vi "Cost Calculation.vi"(5 "Weights":T1={"TS-S weight"=90.0, "CS-S weight"=90.0, "PCS-S weight"=90.0, "Near weight"=90.0, "Mid weight"=90.0, "Far weight"=90.0}, 7 "Previous Calculated Sector":i16=90, 8 "Far Boolean Array":bool[](array[boolean]), 9 "Mid Boolean Array":bool[](array[boolean]), 10 "Near Boolean Array":bool[](array[boolean]), 11 "Target Sector":i16=90) -> (3 "Cost Array":dbl[](array[numeric]))   [LabVIEW 2009]
uses:
  VFH Weights.ctl
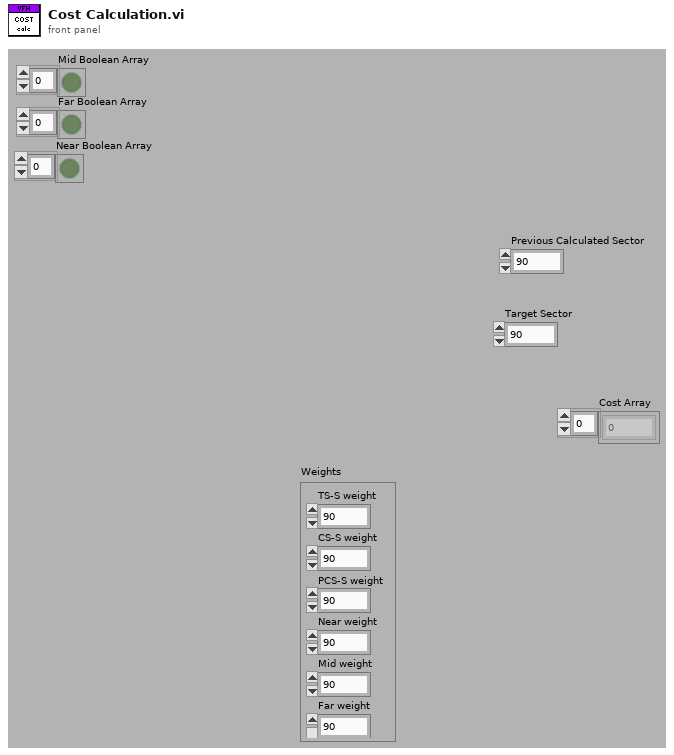
[diagram p1: front panel]
types:
  T1 = typedef "VFH Weights.ctl" = cluster{"TS-S weight":dbl, "CS-S weight":dbl, "PCS-S weight":dbl, "Near weight":dbl, "Mid weight":dbl, "Far weight":dbl}
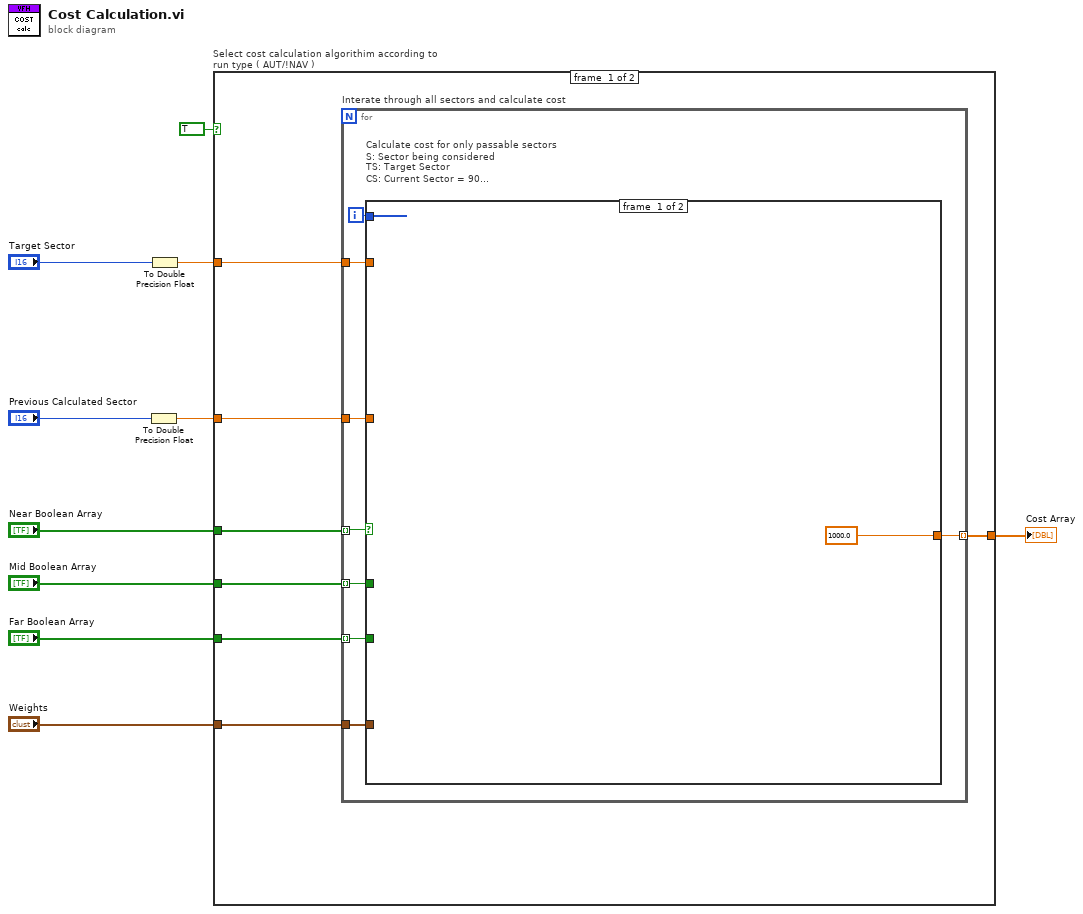
[diagram p0: block diagram]
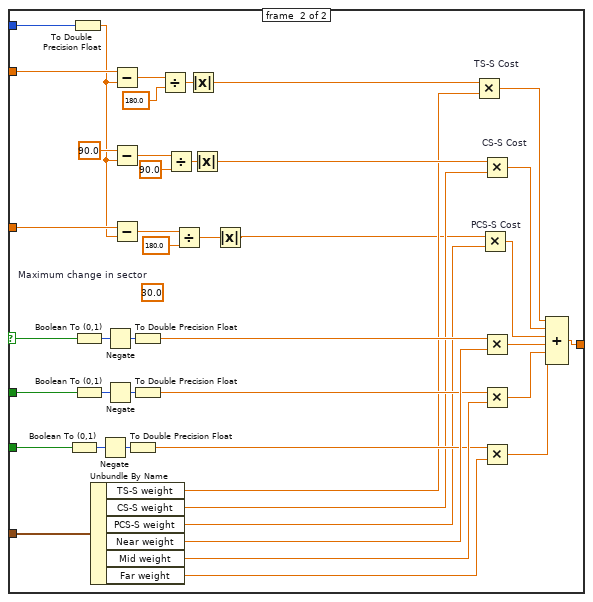
[diagram p2: hidden frame]
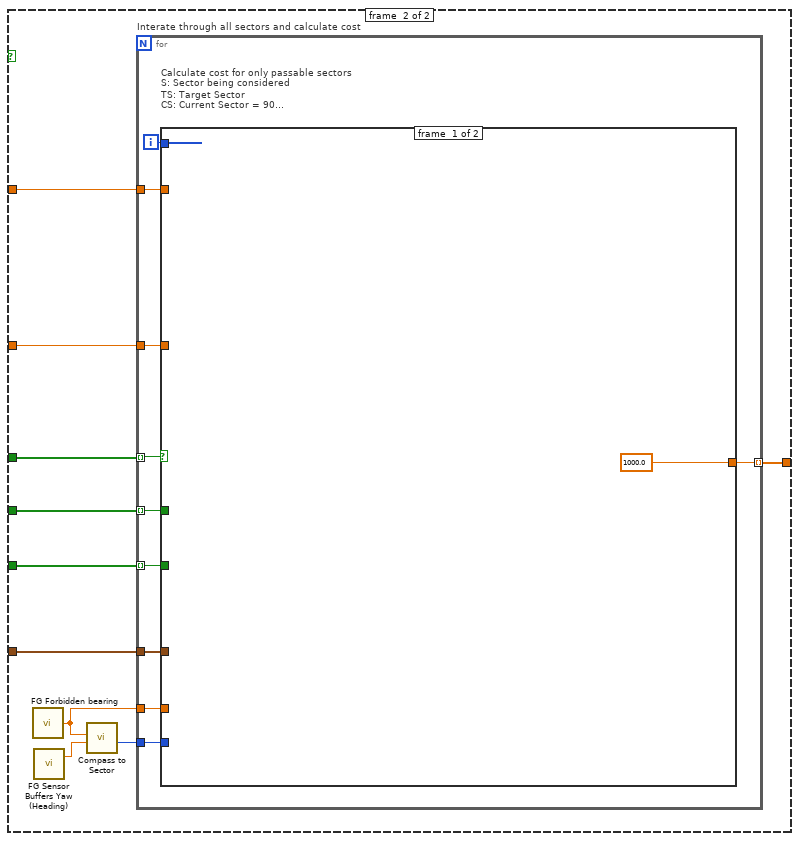
[diagram p3: hidden frame]
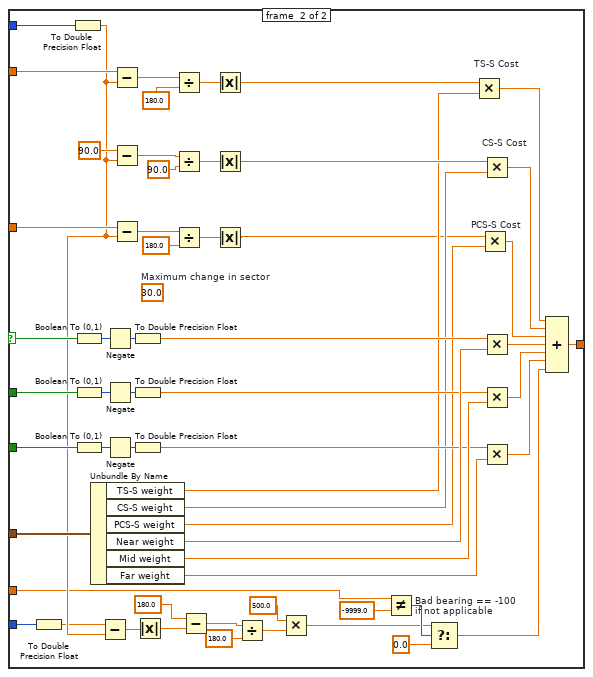
[diagram p4: hidden frame]
diagram:
  n1 = To Double Precision Float(number="Previous Calculated Sector") -> (double precision float=w2:dbl)
  n2 = To Double Precision Float(number="Target Sector") -> (double precision float=w5:dbl)
  n3 = case "Select cost calculation algorithim according to run type ( AUT/!NAV )" shown="True" TRUE {
    tunnel: "Near Boolean Array" -> [w17 w79]
    tunnel: [w16 w78] -> w8
    tunnel: "Mid Boolean Array" -> [w15 w77]
    tunnel: "Far Boolean Array" -> [w14 w76]
    tunnel: w5 -> [w13 w75]
    tunnel: "Weights" -> [w12 w74]
    tunnel: w2 -> [w11 w73]
    frame #0 {
      n4 = for "Interate through all sectors and calculate cost" {
        tunnel: w17 -> [w24] mode=indexing
        tunnel: w13 -> [w20]
        tunnel: [w25] -> w16 mode=indexing
        tunnel: w15 -> [w23] mode=indexing
        tunnel: w14 -> [w22] mode=indexing
        tunnel: w12 -> [w19]
        tunnel: w11 -> [w18]
        i -> [w21]
        n5 = case "Calculate cost for only passable sectors\nS: Sector being considered\nTS: Target Sector\nCS: Current Sector = 90\nPCS: Previous Calculated Sector" shown="True" w24 {
          selector: w24 -> [_ w50]
          tunnel: [1000.0 ("input variable") w53] -> w25
          tunnel: w23 -> [_ w44]
          tunnel: w22 -> [_ w40]
          tunnel: w21 -> [_ w67]
          tunnel: w20 -> [_ w69]
          tunnel: w19 -> [_ w62]
          tunnel: w18 -> [_ w36]
          frame #0 {
          }
          frame #1 {
            (unwired) 30.0  # Maximum change in sector
            n6 = Boolean To (0,1)(Boolean=w40) -> (0, 1=w42:i16)
            n7 = To Double Precision Float(number=w67) -> (double precision float=w35:dbl)
            n8 = Boolean To (0,1)(Boolean=w50) -> (0, 1=w49:i16)
            n9 = Boolean To (0,1)(Boolean=w44) -> (0, 1=w45:i16)
            n10 = Unbundle By Name(w62) -> ("TS-S weight"=w38:dbl, "CS-S weight"=w37:dbl, "PCS-S weight"=w32:dbl, "Near weight"=w59:dbl, "Mid weight"=w58:dbl, "Far weight"=w57:dbl)
            n11 = Negate(x=w42) -> (-x=w41:i16)
            n12 = Negate(x=w49) -> (-x=w48:i16)
            n13 = Negate(x=w45) -> (-x=w46:i16)
            n14 = Subtract(x=w69, y=w35) -> (x-y=w68:dbl)
            n15 = Subtract(x=90.0, y=w35) -> (x-y=w66:dbl)
            n16 = Subtract(x=w36, y=w35) -> (x-y=w28:dbl)
            n17 = To Double Precision Float(number=w41) -> (double precision float=w39:dbl)
            n18 = To Double Precision Float(number=w48) -> (double precision float=w47:dbl)
            n19 = To Double Precision Float(number=w46) -> (double precision float=w43:dbl)
            n20 = Divide(x=w68, y=180.0) -> (x/y=w61:dbl)
            n21 = Divide(x=w66, y=90.0) -> (x/y=w60:dbl)
            n22 = Divide(x=w28, y=180.0) -> (x/y=w29:dbl)
            n23 = Absolute Value(x=w61) -> (abs(x)=w52:dbl)
            n24 = Absolute Value(x=w60) -> (abs(x)=w51:dbl)
            n25 = Absolute Value(x=w29) -> (abs(x)=w27:dbl)
            n26 = Multiply "TS-S Cost"(x=w52, y=w38) -> (x*y=w34:dbl)
            n27 = Multiply "PCS-S Cost"(x=w27, y=w32) -> (x*y=w31:dbl)
            n28 = Multiply "CS-S Cost"(x=w51, y=w37) -> (x*y=w33:dbl)
            n29 = Multiply(x=w47, y=w59) -> (x*y=w56:dbl)
            n30 = Multiply(x=w43, y=w58) -> (x*y=w55:dbl)
            n31 = Multiply(x=w39, y=w57) -> (x*y=w54:dbl)
            n32 = Compound Arithmetic op=ADD(w34, w33, w31, w56, w55, w54) -> (w53:dbl)
          }
        }
      }
    }
    frame #1 {
      n33 = call "FG Forbidden bearing.vi"() -> ("Forbidden bearing out"=w70:dbl)  [unwired: 2 in]
      n34 = call "FG Sensor Buffers Yaw (Heading).vi"() -> ("Yaw Buffer Out"=w72:dbl)  [unwired: 3 in]
      n35 = call "Compass to Sector.vi"("Target Bearing (degrees)"=w72, "Compass Bearing (degrees)"=w70) -> ("Target Heading (Sectors)"=w71:i16)  [unwired: 9 out]
      n36 = for "Interate through all sectors and calculate cost" {
        tunnel: w79 -> [w88] mode=indexing
        tunnel: w75 -> [w84]
        tunnel: [w89] -> w78 mode=indexing
        tunnel: w77 -> [w87] mode=indexing
        tunnel: w76 -> [w86] mode=indexing
        tunnel: w74 -> [w83]
        tunnel: w73 -> [w82]
        tunnel: w71 -> [w81]
        tunnel: w70 -> [w80]
        i -> [w85]
        n37 = case "Calculate cost for only passable sectors\nS: Sector being considered\nTS: Target Sector\nCS: Current Sector = 90\nPCS: Previous Calculated Sector" shown="True" w88 {
          selector: w88 -> [_ w129]
          tunnel: [1000.0 ("input variable") w132] -> w89
          tunnel: w87 -> [_ w123]
          tunnel: w86 -> [_ w119]
          tunnel: w85 -> [_ w146]
          tunnel: w84 -> [_ w148]
          tunnel: w83 -> [_ w141]
          tunnel: w82 -> [_ w115]
          tunnel: w81 -> [_ w106]
          tunnel: w80 -> [_ w96]
          frame #0 {
          }
          frame #1 {
            (unwired) 30.0  # Maximum change in sector
            n38 = To Double Precision Float(number=w106) -> (double precision float=w104:dbl)
            n39 = To Double Precision Float(number=w146) -> (double precision float=w105:dbl)
            n40 = Boolean To (0,1)(Boolean=w129) -> (0, 1=w128:i16)
            n41 = Boolean To (0,1)(Boolean=w123) -> (0, 1=w124:i16)
            n42 = Boolean To (0,1)(Boolean=w119) -> (0, 1=w121:i16)
            n43 = Unbundle By Name(w141) -> ("TS-S weight"=w117:dbl, "CS-S weight"=w116:dbl, "PCS-S weight"=w112:dbl, "Near weight"=w138:dbl, "Mid weight"=w137:dbl, "Far weight"=w136:dbl)
            n44 = Subtract(x=w104, y=w105) -> (x-y=w103:dbl)
            n45 = Negate(x=w128) -> (-x=w127:i16)
            n46 = Negate(x=w124) -> (-x=w125:i16)
            n47 = Negate(x=w121) -> (-x=w120:i16)
            n48 = Subtract(x=w148, y=w105) -> (x-y=w147:dbl)
            n49 = Subtract(x=90.0, y=w105) -> (x-y=w145:dbl)
            n50 = Subtract(x=w115, y=w105) -> (x-y=w108:dbl)
            n51 = To Double Precision Float(number=w127) -> (double precision float=w126:dbl)
            n52 = To Double Precision Float(number=w125) -> (double precision float=w122:dbl)
            n53 = To Double Precision Float(number=w120) -> (double precision float=w118:dbl)
            n54 = Absolute Value(x=w103) -> (abs(x)=w102:dbl)
            n55 = Divide(x=w147, y=180.0) -> (x/y=w140:dbl)
            n56 = Divide(x=w145, y=90.0) -> (x/y=w139:dbl)
            n57 = Divide(x=w108, y=180.0) -> (x/y=w109:dbl)
            n58 = Subtract(x=180.0, y=w102) -> (x-y=w99:dbl)
            n59 = Absolute Value(x=w140) -> (abs(x)=w131:dbl)
            n60 = Absolute Value(x=w139) -> (abs(x)=w130:dbl)
            n61 = Absolute Value(x=w109) -> (abs(x)=w107:dbl)
            n62 = Divide(x=w99, y=180.0) -> (x/y=w98:dbl)
            n63 = Multiply(x=500.0, y=w98) -> (x*y=w92:dbl)
            n64 = Not Equal? "Bad bearing == -100\nif not applicable"(x=w96, y=-9999.0) -> (x != y?=w95:bool)
            n65 = Select(t=w92, s=w95, f=0.0) -> (s? t:f=w94:dbl)
            n66 = Multiply "TS-S Cost"(x=w131, y=w117) -> (x*y=w114:dbl)
            n67 = Multiply "PCS-S Cost"(x=w107, y=w112) -> (x*y=w111:dbl)
            n68 = Multiply "CS-S Cost"(x=w130, y=w116) -> (x*y=w113:dbl)
            n69 = Multiply(x=w126, y=w138) -> (x*y=w135:dbl)
            n70 = Multiply(x=w122, y=w137) -> (x*y=w134:dbl)
            n71 = Multiply(x=w118, y=w136) -> (x*y=w133:dbl)
            n72 = Compound Arithmetic op=ADD(w114, w113, w111, w135, w134, w133, w94) -> (w132:dbl)
          }
        }
      }
    }
  }
  "Cost Array" <- w8
